vi "joe_johnson_map_button_to_state.vi"(10 "Button":bool, 11 "joe_johnson_state":T1=enum."down") -> ()   [LabVIEW 2011]
uses:
  joe_johnson_state.ctl
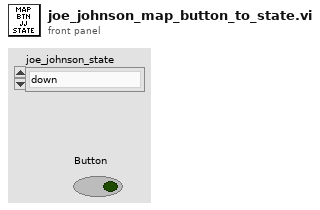
[diagram p1: front panel]
types:
  T1 = typedef "joe_johnson_state.ctl" = enum16{"fold", "down", "up", "ramp", "bridge_lift", "manual", "ramp_stay"}
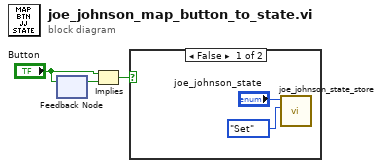
[diagram p0: block diagram]
diagram:
  n1 = feedback-in #1("Button") -> ()
  n2 = feedback #1() -> (w2:bool)  [unwired: 1 in]
  n3 = Implies(1:w2, 2:"Button") -> (0:w1:bool)
  n4 = case shown="False" w1 {
    frame False {
      n5 = call "joe_johnson_state_store.vi"("data_store_mode"=enum16{"Set", "Get"}."Set", "joe_johnson_state"="joe_johnson_state") -> ()  [unwired: 7 in, 3 out]
    }
    frame True {
    }
  }
